vi "Read configuration.vi"(8 "error in (no error)":errorcluster, 11 "Instrument Device in":refnum<class "Switch Instrument.lvclass">) -> (0 "error out":errorcluster, 2 "configuration":refnum<class "CEF_serializable configuration.lvclass">, 3 "Instrument Device out":refnum<class "Switch Instrument.lvclass">)   [LabVIEW 2025, in "Switch.lvlib" / "Switch Instrument.lvclass"]
uses:
  Switch Instrument.lvclass
  Users/Public/Documents/Sandia National Labs/TSS Plugin/CEF.lvlibp/serializable configuration/CEF_serializable configuration.lvclass
  Switch Instrument.lvclass/Switch Instrument.ctl
  Users/Public/Documents/Sandia National Labs/TSS Plugin/Abstract PlugIn.lvlibp/Plugin/Abstract/Instrument configuration/Instrument configuration.lvclass
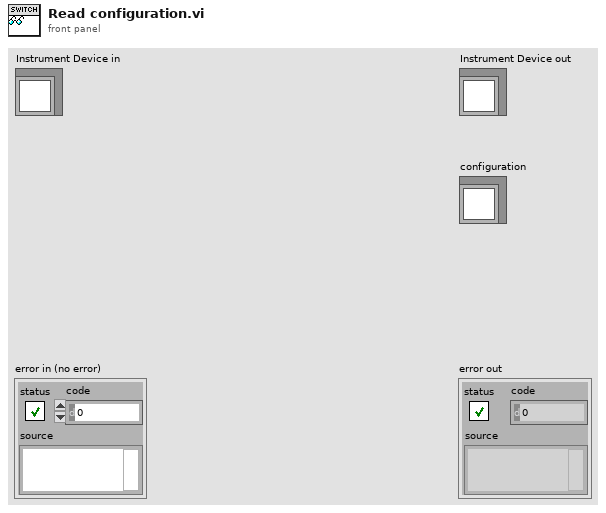
[diagram p1: front panel]
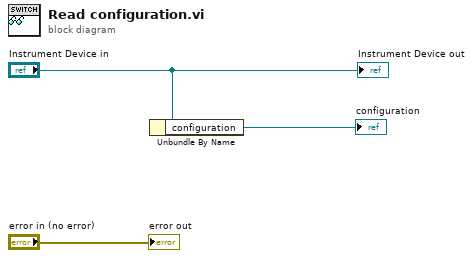
[diagram p0: block diagram]
diagram:
  n1 = Unbundle By Name("Instrument Device in") -> ("configuration"=→"configuration":refnum<class "Instrument configuration.lvclass">)
  "error out" <- "error in (no error)"
  "Instrument Device out" <- "Instrument Device in"
